vi "20_1.vi"() -> ()   [LabVIEW 2020]
uses:
  Tile/Tile.lvclass
  Tile/Set Tile ID.vi
  Tile/Set Tile.vi
  Tile/Get Matching Sides.vi
  <userlib>/_OpenG.lib/array/array.llb/Search 1D Array (U64)__ogtk.vi
  <userlib>/_OpenG.lib/array/array.llb/Index 1D Array Elements (U64)__ogtk.vi
panel:
  out "product":u64=8425574315321
  out "elements":u64[](array[numeric])=[1153, 1163, 1619, 3881]
  in  "Switch":bool
  in  "Input":string="Tile 3571:\n##..##....\n..##..#..#\n#...##....\n.....#...#\n..........\n...###....\n#......##.\n#...#...#.\n#...##...#\n#.####.##.\n\nTile 2687:\n#..##..###\n..........\n.....##..#\n.#.#..##.#\n#.#..#..##\n#.....#...\n#...#.....\n##....##..\n#...#...##\n..#.#.#.##\n\nTile 3049:\n##.#.#.###\n....##.###\n....##....\n#.........\n#.#...#..#\n#..##....#\n#.#......#\n#..#..##..\n#......###\n#.#..#...#\n\nTile 1597:\n###..##...\n##.....###\n.#..#..#.#\n#.......#.\n#.#.......\n.#..#.....\n#.....#...\n#........#\n##.#...##.\n.....#.###\n\nTile 1301:\n#.##.#.###\n#........#\n....#.....\n#.....####\n.#....#.##\n.....#....\n#..##..#.#\n.....#..##\n.#.##..#.#\n#...######\n\nTile 3259:\n..#####.#.\n.....#...#\n#...#.....\n...##...#.\n.#..#..##.\n.#.......#\n........##\n#.......#.\n.#.#...#..\n#...#.#..#\n\nTile 3989:\n#..#..####\n..........\n#........#\n.#....#...\n..........\n#.........\n.#........\n#........#\n...##.####\n.######.##\n\nTile 3803:\n#.####...#\n.###.#..#.\n....##..#.\n#........#\n..##..#...\n####.#....\n..#...#...\n#..#.....#\n..##....#.\n#....#...#\n\nTile 2897:\n.#..##.#.#\n..#.#...##\n#........#\n###.#..#.#\n...#..#.##\n...#....##\n....##...#\n.....##..#\n.#....#...\n..##....##\n\nTile 2843:\n##.###..##\n#.#.......\n#....#....\n#..##.##..\n.##..#.##.\n#....#....\n#.#...#.##\n..........\n.#...#...#\n###..#..##\n\nTile 3023:\n.#..###.#.\n.........#\n..........\n.#........\n#.#....#.#\n....#...#.\n#.......#.\n##.#.....#\n..#...#..#\n.....####.\n\nTile 2887:\n#....##...\n#...#.....\n##...##...\n#.....##.#\n.......#..\n#......#.#\n..##..#..#\n....#....#\n#.###.....\n#.####..#.\n\nTile 1013:\n#..####.#.\n#.##...#.#\n#..#..#...\n#..#..#..#\n...#......\n#.####...#\n.#..##..##\n...#.#..##\n....##..##\n#.##.#.#.#\n\nTile 3733:\n###.##.#.#\n..#....#..\n#...#.#..#\n....###..#\n.#........\n.....#....\n........##\n##........\n#........#\n#.#...#..#\n\nTile 3691:\n.##...####\n##..##....\n#.#.##..##\n#........#\n#.....##.#\n.....#....\n##.#.....#\n#..#.....#\n..#.......\n####....#.\n\nTile 3061:\n##.....#..\n.....#...#\n....##...#\n###.#.....\n#..#..###.\n#.#.###..#\n..#......#\n#..#.#...#\n..#.......\n..#.#..#..\n\nTile 1489:\n###.......\n.....##...\n..#...##..\n#.....#...\n#.#......#\n##.#..####\n...##.#...\n...#...#.#\n..........\n.##.##.#.#\n\nTile 1637:\n#########.\n.#.....#..\n#........#\n#........#\n.##.....##\n.........#\n#....#..##\n#.....####\n...###...#\n.#..##..##\n\nTile 1069:\n#.#...####\n##...#...#\n.....#...#\n.......##.\n......#..#\n#........#\n#...#.....\n......#...\n#.#..#....\n####.##.#.\n\nTile 1039:\n#..#######\n###.......\n.....#....\n#.........\n....#....#\n...####...\n.#...##...\n#.#....#.#\n........##\n#.#..#..#.\n\nTile 2767:\n.#.#..#.##\n.#..#....#\n#..#.#....\n#.#..##..#\n.####.#.##\n#....##...\n....##..##\n###.....#.\n..........\n....#.###.\n\nTile 2957:\n####.#####\n.......##.\n...#.....#\n...##..##.\n...##.##..\n#..#..#..#\n.....#....\n#..#....#.\n.##.......\n.##..#.##.\n\nTile 2789:\n.##..#.#.#\n#.#.....##\n#....#...#\n#....##...\n..#..#....\n#.........\n#.#..#..##\n#........#\n.#.......#\n#####...##\n\nTile 2837:\n.....#...#\n.....#.#.#\n#.......#.\n#...#...#.\n..#.....#.\n..#.#..#..\n##.......#\n....#....#\n#...#.....\n##.###....\n\nTile 3251:\n.######...\n...#......\n.#.#..###.\n#..#.##..#\n###.#....#\n#.#......#\n..#..###..\n##.#..#..#\n...#...###\n##.#..##..\n\nTile 3137:\n#####.#..#\n#.#..#.##.\n#.#..#....\n#.........\n.........#\n.........#\n...#......\n#...#...#.\n....#..#.#\n.#.###.#.#\n\nTile 3433:\n.##..####.\n...#......\n#..##....#\n....#....#\n#..###....\n..#......#\n.#..###...\n.##.#.....\n.........#\n.....#....\n\nTile 2551:\n#.########\n#.#.......\n##..#...##\n#.#..###.#\n#........#\n.#.#....#.\n#........#\n.##....#..\n#........#\n##..##.#..\n\nTile 2647:\n..####..##\n##....#..#\n#.........\n###.#.....\n#......#..\n....#...##\n.#..##.#.#\n.#.#..#...\n.....##.##\n.#.#...#..\n\nTile 1087:\n#..###..##\n#...#.#.#.\n.......#..\n..#.#.#..#\n#.......#.\n#....#....\n....#....#\n##...##..#\n#..#......\n.#..#.###.\n\nTile 1423:\n..#....#.#\n#........#\n.#.##.##..\n#.###.#.#.\n#.#......#\n...##...##\n#....#....\n....#....#\n.........#\n#####....#\n\nTile 1759:\n..#.#..#..\n##...#...#\n....#..#..\n#....#....\n.##..##..#\n...#.#...#\n#..#.....#\n##.......#\n......#..#\n#.##......\n\nTile 1583:\n.###.####.\n......###.\n......#..#\n.#...##...\n#...#....#\n..#.##....\n#...##..#.\n......#...\n#.....###.\n####.#....\n\nTile 1171:\n###......#\n#...##...#\n#####..##.\n#.......#.\n#.#...#..#\n#....#....\n....#....#\n##.....#.#\n#.#..#..##\n#.#.#..##.\n\nTile 2801:\n.###.####.\n......#...\n##..##.#.#\n.....#....\n#......#..\n###..##..#\n##.#..##.#\n#..#..#...\n#..#.#...#\n#..###.###\n\nTile 1559:\n.##..#...#\n#.##..#...\n...##..#..\n..#.#.....\n...#...#..\n.........#\n...#.....#\n#..##.#..#\n##..##....\n...###...#\n\nTile 2609:\n##.#..####\n..........\n#........#\n##.###...#\n#.#..#....\n..#..##..#\n#....#.#.#\n#.#.......\n#....#...#\n#.####.#.#\n\nTile 2287:\n#......#.#\n.....#.#.#\n..#..#...#\n##.#..#...\n..#..#.###\n.......###\n#......##.\n#.##.##...\n......#..#\n#####.##.#\n\nTile 3659:\n.###.#####\n#.#.......\n..........\n..#.....##\n#..#......\n#.#.#...##\n#.........\n.#...#....\n##.....#..\n#####.##.#\n\nTile 3539:\n.......#.#\n..##...#..\n.....#.#.#\n##.#......\n####......\n...#..#...\n#.......##\n#...#.....\n#..#.....#\n.##.#....#\n\nTile 3121:\n..##.#...#\n.###..#...\n##.#.#....\n#.....#..#\n#.#.......\n#.........\n....#...##\n......###.\n#........#\n#..###..##\n\nTile 2237:\n...##.....\n..........\n...#......\n#....#...#\n#.........\n.......#..\n#...###..#\n.....#...#\n.........#\n#.####.##.\n\nTile 1277:\n.###...##.\n.......###\n#.....##..\n#.##..###.\n#.#..#....\n.....#....\n#...#....#\n#.#......#\n#...###..#\n...##...##\n\nTile 2161:\n..#####..#\n#....##..#\n#.....#..#\n....#....#\n.....#.##.\n..........\n#......#.#\n#..#......\n#....#..##\n.##.....#.\n\nTile 3709:\n.#..#...##\n#..#.....#\n...#....#.\n..........\n.#...#....\n..........\n....##....\n#.........\n.........#\n..####....\n\nTile 1117:\n##.##.#..#\n.....##...\n.#.#..#.##\n.#...#..#.\n#.##.#....\n####.....#\n##..#.....\n#.........\n#...##...#\n####..#.#.\n\nTile 2081:\n##.##.###.\n#...#.....\n#.....#...\n#.#..#.#..\n#.....#..#\n...#.....#\n#....#....\n......#..#\n.#.##..#..\n###..#.#.#\n\nTile 1709:\n##...#.##.\n###..#....\n#.......#.\n#.....##..\n.........#\n#....#..##\n..#...##..\n#...#.....\n#...#.#..#\n.###.#....\n\nTile 2927:\n...###..##\n##.#......\n..........\n##........\n#....#...#\n.......##.\n#.....#..#\n##.#.#....\n#......#..\n...#.####.\n\nTile 1499:\n#....##.#.\n......#...\n#........#\n......#...\n.#.......#\n#.#...#.##\n..#....#.#\n#...#.....\n.........#\n#.....##.#\n\nTile 1453:\n#.##.####.\n..#...##..\n.........#\n.........#\n#..#..#...\n.........#\n#....#.#..\n#.....#..#\n.#........\n#....#....\n\nTile 1283:\n.#.##..###\n..#...#.#.\n...##..#..\n#.......#.\n#......#..\n#..##.....\n#.......##\n....##...#\n..#.....##\n##.#.#...#\n\nTile 2063:\n......#.##\n.........#\n....##..#.\n.#....##..\n##........\n.###.###.#\n#.#....#..\n....#...#.\n#......###\n#....####.\n\nTile 3529:\n...###.##.\n#....#...#\n...#.....#\n...#.#..#.\n.#.#.....#\n#...#.....\n##..#..#..\n#.....#..#\n.#........\n.#..#####.\n\nTile 2657:\n..#.##..#.\n##..#...##\n#.....#...\n#....##...\n.....#..##\n#.#..##.##\n#.........\n#.#...##.#\n##....#...\n##..####.#\n\nTile 2089:\n.#########\n##.#.##..#\n#........#\n#..###..##\n...#......\n##..#....#\n#...#..#..\n#..#....#.\n..#.#....#\n...###...#\n\nTile 3779:\n#.#...##.#\n.##...##..\n.....##...\n.#....##.#\n###..##..#\n#.#..#.#..\n....##...#\n##...#....\n.#...#....\n#######...\n\nTile 3217:\n...##.....\n....##....\n.....##..#\n##...#.#.#\n###.......\n...#...#..\n...#.....#\n#..#.#.###\n##.#...#.#\n.#.#..##..\n\nTile 3907:\n..#..##.##\n#.#.....##\n#.......#.\n.#...###..\n..###.####\n##.#..##..\n#.........\n##...#..#.\n#....#....\n.#.....#.#\n\nTile 3547:\n#..#.##...\n#..###...#\n##.......#\n.....#....\n#...#...#.\n#..#..#...\n........#.\n......##.#\n.......#..\n.##.#..##.\n\nTile 3187:\n##.#.##...\n#...#.##.#\n#...#.....\n#....#..##\n....#.#..#\n.....#....\n.....#..##\n....##...#\n..........\n#######.##\n\nTile 1217:\n##.#####..\n#.......#.\n...#....##\n#........#\n#.#......#\n.....#...#\n#.........\n....#...##\n#...#.....\n.#...###.#\n\nTile 3821:\n#.###.###.\n#.#......#\n#..#.#...#\n.##...#.##\n...#....##\n#...#..##.\n#......#.#\n###..#...#\n.........#\n#....##.##\n\nTile 1607:\n##..#..##.\n#.##....##\n###.##.##.\n.#....##.#\n#.#..#...#\n.....#.#..\n#.#..#..#.\n#.#..#....\n..........\n......##.#\n\nTile 1459:\n.###.##..#\n#.......#.\n##........\n..#...####\n###.......\n#....#....\n.#.....#.#\n###..#..##\n.....#....\n..#..#..##\n\nTile 2129:\n....#.#..#\n#.....##.#\n#........#\n..........\n..#......#\n#.....#..#\n.#..##...#\n#.#.#..#.#\n#.........\n#.##....##\n\nTile 1601:\n.#.#.#.#.#\n..#..##...\n#.#.#...#.\n....##....\n....##.#..\n..#.......\n#.....#..#\n#..##.#...\n.........#\n...####.#.\n\nTile 1801:\n#.#...#.#.\n..#....#..\n#..#...#..\n......#...\n.....#....\n#.#..##.##\n#.........\n...#.#...#\n.#....#..#\n#.....##..\n\nTile 2447:\n..#.....##\n.#..#...##\n.....#.#..\n.#....#..#\n#...####.#\n##.##..###\n.#.......#\n#.##.....#\n#.......##\n.###.#...#\n\nTile 2203:\n#.....##..\n#.#.......\n........##\n###...#...\n..........\n#..#.....#\n....#.##.#\n..##.....#\n.#...#...#\n#.###..#..\n\nTile 1381:\n.#...#...#\n....#.....\n##.......#\n#.....#...\n.........#\n.#.......#\n.......##.\n#.#.....##\n.#..#.##..\n##.#.##.#.\n\nTile 3163:\n#...####.#\n#......##.\n...###.#.#\n#....##...\n#......###\n.....#..##\n.#..###...\n#..##..#..\n#.....#...\n#.#####.##\n\nTile 3673:\n.#....##.#\n..#..####.\n#.....#...\n...#....#.\n#....#...#\n#....##.#.\n##...#.#..\n.#..#.#...\n#..#.....#\n####.##...\n\nTile 3919:\n....##.##.\n##..##....\n...##...##\n#...#.....\n..........\n....#..###\n.#.....#..\n....#..#.#\n.##..#....\n.#...###.#\n\nTile 2437:\n..##...#.#\n#....#...#\n#..#.....#\n..#.#...##\n.......#..\n........##\n........##\n.......#.#\n#....#.#.#\n##..#.###.\n\nTile 2969:\n##.#.##.#.\n#.##....#.\n.##......#\n#.#.#....#\n#.#.......\n.........#\n....#.#.##\n.#.......#\n...#..#.##\n##.#.##..#\n\nTile 2621:\n.##.##.#..\n.##...#...\n..........\n#.........\n#.#.#.#..#\n..#..#...#\n.......#.#\n#.#.....##\n...#..#...\n#.......##\n\nTile 3613:\n##..#....#\n#..##.....\n..#.......\n..#...#...\n...#...#..\n...#.....#\n..#.....#.\n..#.###..#\n..........\n..#.####..\n\nTile 2777:\n##.#####.#\n#.##.#...#\n..#.......\n.##...##.#\n.........#\n.#.###.##.\n#......##.\n#......##.\n#...##..##\n#..#....##\n\nTile 2711:\n#..#..##..\n..........\n#.#......#\n#.....####\n..........\n##.......#\n........#.\n#.......#.\n#.#..#...#\n#.#.####.#\n\nTile 2281:\n.#.###...#\n###....#..\n..........\n#.#..#..##\n.........#\n###..#.##.\n####..#..#\n##..#.....\n##..#..#..\n#.....#..#\n\nTile 1579:\n....#..#..\n#........#\n#...#..#..\n..##.#.#..\n.###.#...#\n....##..#.\n...##.#...\n.#.##....#\n.#.......#\n##...#...#\n\nTile 2411:\n#.#....##.\n..#...#..#\n.#..##....\n.#..##...#\n.....#.#.#\n......##..\n#.#....###\n.#.##....#\n..#..#....\n..#.###..#\n\nTile 2963:\n.......##.\n.....#....\n.........#\n#.....#..#\n.....#.#..\n.....#.##.\n.#.#...###\n#.#.......\n.#.......#\n###..#..#.\n\nTile 1693:\n#.##..##..\n..........\n.........#\n.##..#...#\n.........#\n#........#\n###......#\n..#...#...\n.#.##....#\n...#.#...#\n\nTile 2399:\n###.#.##..\n#...#.....\n...#...#.#\n###.......\n.##.##....\n##.....#.#\n####......\n##.......#\n#..#...#.#\n#...#.....\n\nTile 1913:\n##.....###\n........##\n#.....###.\n..........\n....#...#.\n#.#.....#.\n#....#...#\n..#...#...\n....#..#..\n#..####...\n\nTile 3343:\n.....#.##.\n..#...#...\n####.....#\n....#.....\n......#..#\n......#...\n#........#\n#.......#.\n..#...#.#.\n.....###.#\n\nTile 2557:\n#.......##\n....#...##\n#......#.#\n#.#.#.#.##\n#..##.....\n..###.#.#.\n#..#......\n#...#.....\n....#....#\n#.##...#.#\n\nTile 1097:\n.#.#.#..##\n..#.#.....\n##........\n.##...##..\n..#..#...#\n#........#\n........##\n#.#.#.....\n.#.#.....#\n#.##..#...\n\nTile 2591:\n##..#..###\n......#...\n...###.#..\n#.......#.\n#.#.....#.\n#.##..#...\n....##.#..\n#.#..#...#\n#.###..#.#\n##........\n\nTile 3413:\n...##...##\n..#....#..\n##.#....#.\n#..#....#.\n#........#\n#..#......\n#.....#.##\n##.....#.#\n#....#....\n####.#...#\n\nTile 2087:\n###..###.#\n##......#.\n#..#...#.#\n#.#.......\n##.#.....#\n#.#.#.....\n...#.....#\n..........\n#.........\n#.##..###.\n\nTile 3037:\n......##..\n..#..#....\n#.#.......\n#.#....#..\n.#.#.##..#\n#.....#.##\n#.....#.#.\n.#..##...#\n#....##...\n...#..###.\n\nTile 2239:\n.####..#..\n#.........\n.#.......#\n#..##.....\n##..##..##\n#.#....#..\n.........#\n#.......#.\n....#.....\n#.###..#.#\n\nTile 3313:\n##.##.#..#\n.#.#..#...\n.##...##.#\n.#.##..#..\n##........\n..........\n#..#.#....\n#.........\n..........\n.##..#..#.\n\nTile 3361:\n.###.#...#\n##..#.#..#\n...##....#\n#..##.....\n..........\n#......#.#\n.........#\n..#..##.#.\n#..#...###\n#...#.#.#.\n\nTile 3167:\n..##..####\n#.....#.#.\n.....#.#..\n...#......\n....#.#.##\n...#.#.#..\n.......#..\n##........\n#..#...#.#\n####.##..#\n\nTile 1979:\n#.#.###...\n..#.....##\n...#...##.\n#.......##\n........##\n..##..#...\n..#......#\n#.#....#.#\n#..#.....#\n.##.......\n\nTile 1831:\n##.##.##.#\n#.........\n.........#\n##.......#\n###.....##\n..##..##..\n##.....#.#\n#....#...#\n###.##..#.\n#..#####..\n\nTile 1487:\n#..#....##\n.#..#....#\n#....#....\n#.........\n#.#...#.##\n#..##...##\n...##..#..\n.#...##...\n.#........\n.#...#..#.\n\nTile 1987:\n###..#....\n##..##...#\n......#..#\n.#.#...#.#\n.....#.#..\n....#..#..\n....###..#\n#...##....\n###.....#.\n...##.####\n\nTile 3083:\n....##..#.\n##..#.###.\n#..#...##.\n#.###.....\n.........#\n....#.....\n.#........\n.#........\n#.........\n#.#.#.##.#\n\nTile 1543:\n...##..###\n.........#\n.......#.#\n#..#..#.##\n##....#.#.\n....#..#..\n#..#......\n...#...#.#\n##.##..#..\n#.###..#..\n\nTile 1151:\n#.#..#####\n#.#..#...#\n#..#......\n....#...#.\n..........\n#...#.#..#\n#..#.#...#\n##....#..#\n#.........\n##.....###\n\nTile 1009:\n##..#...##\n#....#...#\n.#...#....\n#........#\n.#..#..#..\n.###.##.#.\n#......#.#\n##.#..##..\n#....#.###\n####...##.\n\nTile 3929:\n......#.#.\n#..#.##.##\n....#.#.##\n#.##..#...\n###..#..#.\n.##..###.#\n.##......#\n....#....#\n........#.\n.#...###..\n\nTile 1321:\n#.##..#...\n.##.....##\n#.#..#....\n...#.....#\n###......#\n#.#.#.##.#\n##.......#\n##......#.\n.#...#....\n.#..##..##\n\nTile 2017:\n###.#..###\n.#..###..#\n#..#......\n.........#\n..#...##..\n....#.##.#\n...##.#..#\n....#...##\n#..#..##..\n##.#.#.#..\n\nTile 1747:\n....##.#..\n#........#\n.....#..#.\n..#####...\n######..#.\n##..#.#...\n.###..#..#\n#.....#...\n.##..#..##\n..#####...\n\nTile 3089:\n#....#.##.\n#.....#..#\n..........\n#..#.#....\n.......#..\n#.....#...\n........#.\n##..#..##.\n#.....#..#\n#.#.#....#\n\nTile 3019:\n.#..###.##\n.#...#...#\n#.#.......\n###.......\n#....#...#\n#.##...#..\n##........\n.#.......#\n.#.#......\n.#..#...#.\n\nTile 3079:\n...#.###..\n#......#..\n#.......##\n#...#..###\n#.......#.\n......#.#.\n#........#\n.#.#...###\n..#.#....#\n...#...#.#\n\nTile 1663:\n##.##..###\n#.....##.#\n......#.##\n#........#\n..#.#.....\n....#..#.#\n#.#.#..#.#\n#.......#.\n..#......#\n#.#..#....\n\nTile 1823:\n.###...###\n#.#.#..##.\n..........\n.........#\n###....#..\n..........\n##....#.##\n#.......##\n..#..#...#\n......####\n\nTile 3823:\n....#..#..\n..#.#..#.#\n###.#.##.#\n..##....#.\n#.........\n#....#...#\n#.......##\n#.#...##..\n..#....#..\n..#....##.\n\nTile 1901:\n#.#.#....#\n..#....#.#\n...#..#.#.\n.#..#..###\n....####..\n......#...\n#....#....\n..#....#..\n#......#..\n######.#..\n\nTile 3347:\n#.#.....#.\n#..#..#...\n#.#.......\n#..#.#....\n...#......\n#.........\n##.#.....#\n#........#\n#....#...#\n#.#.##.###\n\nTile 1873:\n..###.#.##\n.#.#....#.\n#........#\n..#..#...#\n##.....#..\n#........#\n#.........\n.#........\n#.#..#.#.#\n.##.#...##\n\nTile 2053:\n#.#.#.#..#\n#...###..#\n##.##.##.#\n....##.#.#\n#.###....#\n#.....#..#\n#..##.####\n....#..#..\n#.........\n#..#.#..#.\n\nTile 2659:\n.#....##.#\n#.#......#\n#..#......\n.#.###.#.#\n..........\n#........#\n.......#.#\n....#....#\n#........#\n##..##.#..\n\nTile 2503:\n.#..####.#\n#.##......\n..#....###\n..#..#.###\n...##...##\n..#.....#.\n..........\n##.#......\n#.#.......\n#...#..#.#\n\nTile 3881:\n##.###.###\n#......#..\n#...#....#\n..#.#....#\n#..#..#..#\n#..#.....#\n...#..##.#\n#.#.......\n#..##....#\n...#.##...\n\nTile 1973:\n..#.###.#.\n#.##....##\n#.......##\n##......##\n#.........\n#.#..#....\n.#....###.\n..#.#..#..\n......#..#\n#..#.....#\n\nTile 3329:\n.#.#.###.#\n..#.#.....\n.#.......#\n#..#.##.##\n#.##..####\n..#.##..##\n....#.....\n#...#.#.#.\n...#.#...#\n.#...##..#\n\nTile 3331:\n#......###\n#......#.#\n#.#.#.#..#\n........#.\n.##.####..\n#..#..#..#\n.#.......#\n......#.##\n......#.#.\n.##...#.#.\n\nTile 1307:\n##.#.#..#.\n.........#\n.#....##.#\n#.........\n#.........\n#....#.#..\n........##\n......##..\n..#.##...#\n..##...##.\n\nTile 2543:\n.#.#.##.##\n#........#\n..##......\n#.........\n##...#...#\n.###..##.#\n.##......#\n.#........\n.....#.#..\n...######.\n\nTile 2003:\n#.#..#.#.#\n.....#....\n#.#.#.....\n####.#..##\n..###....#\n....#.#...\n#.####...#\n.##...#.##\n#.#.#..#..\n...#.....#\n\nTile 3301:\n##....##.#\n.....#...#\n#........#\n..........\n###.##.#..\n.....#...#\n#.#......#\n....##...#\n#........#\n.#.#...#.#\n\nTile 2297:\n#..#.##..#\n...#.#.##.\n..###..#..\n##..#.....\n####..#..#\n..#.#..#..\n.....#...#\n#...#.....\n#.....#..#\n##....#...\n\nTile 2311:\n##.....#.#\n##........\n#........#\n#...##....\n#......#..\n.........#\n.........#\n#..#.#....\n.....#...#\n###.#..##.\n\nTile 1361:\n.#.##.#..#\n#.#..#...#\n#....###..\n..###.#...\n#..#.....#\n#..#...##.\n#.#.....#.\n.......#.#\n##.##.....\n#.###.#..#\n\nTile 1481:\n.####.#.##\n..........\n.........#\n###.#.#...\n##....##.#\n..#...#.##\n..##.#.#..\n#.#.....##\n.......#..\n....###...\n\nTile 1153:\n.##.##..##\n###......#\n#....##...\n......#.#.\n#....#....\n.....##..#\n.....#...#\n#.........\n#...#....#\n##..#.#...\n\nTile 2153:\n#.###.#..#\n..#.##....\n..##....#.\n##...#...#\n#...#.....\n........#.\n#..##...#.\n..#.......\n#...##.#..\n#.#.#.#...\n\nTile 2377:\n.##..##.#.\n...##..#.#\n#.#.#.....\n#.##......\n#.....#..#\n#...#....#\n...##....#\n...###....\n.#.##...##\n.###.##...\n\nTile 3863:\n.##.###.##\n.......#.#\n#........#\n##.#.#...#\n##...#...#\n#...##....\n#..#..#.##\n.....#####\n##.#..###.\n....###...\n\nTile 1163:\n##..######\n#........#\n.#.#...###\n..#..#...#\n##..#...##\n#.#.......\n#.#..#....\n#..#.#....\n###..#...#\n.#####.###\n\nTile 2207:\n.#..#.#.##\n##.....#.#\n#..#.....#\n#..#....##\n.........#\n...#.....#\n#...#..#..\n..#.....##\n.....#....\n#.##.....#\n\nTile 1201:\n#.##.##..#\n#.#.......\n#..#.....#\n.###...#..\n#.#......#\n........##\n.........#\n.##....#.#\n..##.#...#\n.......###\n\nTile 1619:\n#.....#.#.\n...#.##..#\n#.....#...\n#...#.....\n#..#...#.#\n#..##.#...\n.#...#.#..\n#......##.\n#.........\n#.##...###\n\nTile 3389:\n...#..##..\n#........#\n#...#.....\n#.#....#.#\n###....#.#\n#.#....###\n#..##..#.#\n.##.#.#..#\n#...###...\n#...#....#\n\nTile 3359:\n.###..##..\n#........#\n###...#.#.\n........##\n....#..#.#\n.#.#......\n#........#\n.......#.#\n.#.....#..\n##.###....\n"
  in  "Input Test":string="Tile 2311:\n..##.#..#.\n##..#.....\n#...##..#.\n####.#...#\n##.##.###.\n##...#.###\n.#.#.#..##\n..#....#..\n###...#.#.\n..###..###\n\nTile 1951:\n#.##...##.\n#.####...#\n.....#..##\n#...######\n.##.#....#\n.###.#####\n###.##.##.\n.###....#.\n..#.#..#.#\n#...##.#..\n\nTile 1171:\n####...##.\n#..##.#..#\n##.#..#.#.\n.###.####.\n..###.####\n.##....##.\n.#...####.\n#.##.####.\n####..#...\n.....##...\n\nTile 1427:\n###.##.#..\n.#..#.##..\n.#.##.#..#\n#.#.#.##.#\n....#...##\n...##..##.\n...#.#####\n.#.####.#.\n..#..###.#\n..##.#..#.\n\nTile 1489:\n##.#.#....\n..##...#..\n.##..##...\n..#...#...\n#####...#.\n#..#.#.#.#\n...#.#.#..\n##.#...##.\n..##.##.##\n###.##.#..\n\nTile 2473:\n#....####.\n#..#.##...\n#.##..#...\n######.#.#\n.#...#.#.#\n.#########\n.###.#..#.\n########.#\n##...##.#.\n..###.#.#.\n\nTile 2971:\n..#.#....#\n#...###...\n#.#.###...\n##.##..#..\n.#####..##\n.#..####.#\n#..#.#..#.\n..####.###\n..#.#.###.\n...#.#.#.#\n\nTile 2729:\n...#.#.#.#\n####.#....\n..#.#.....\n....#..#.#\n.##..##.#.\n.#.####...\n####.#.#..\n##.####...\n##..#.##..\n#.##...##.\n\nTile 3079:\n#.#.#####.\n.#..######\n..#.......\n######....\n####.#..#.\n.#...#.##.\n#.#####.##\n..#.###...\n..#.......\n..#.###..."
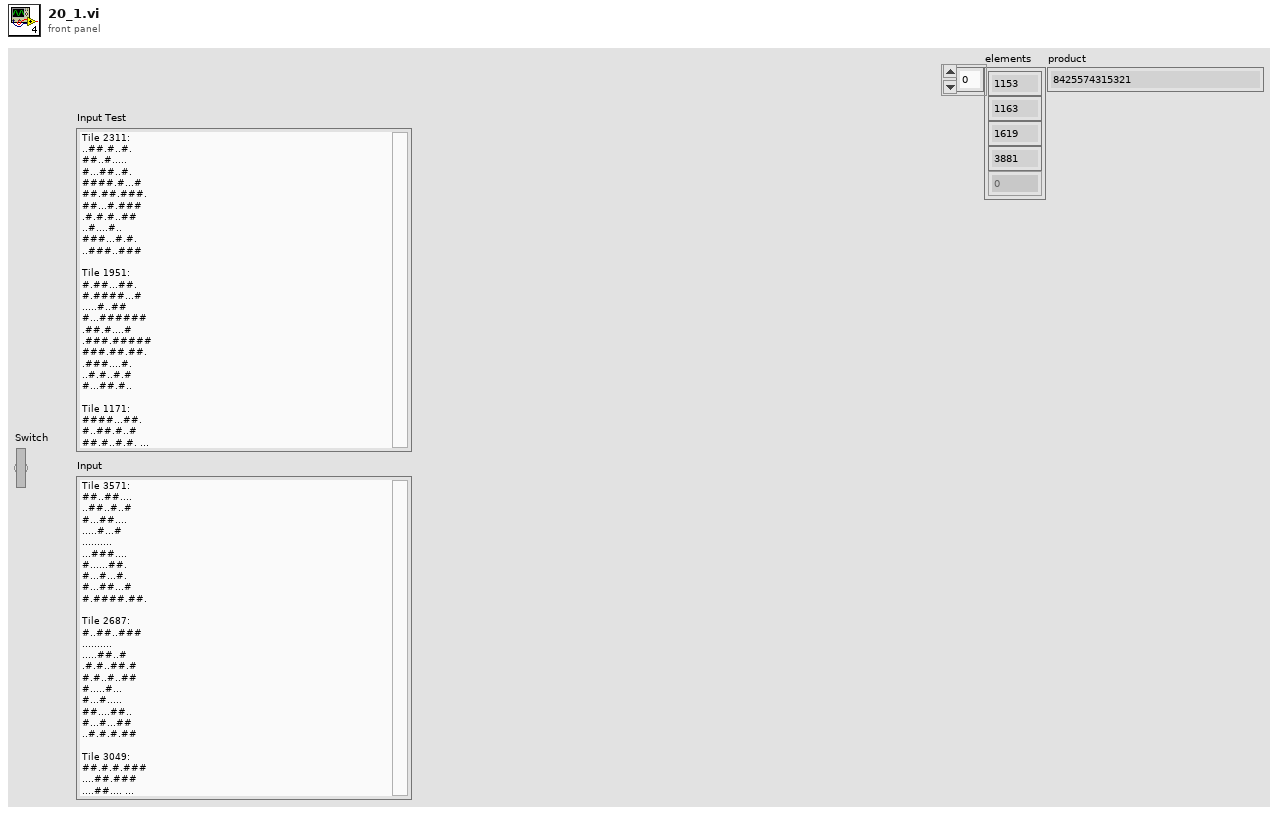
[diagram p1: front panel]
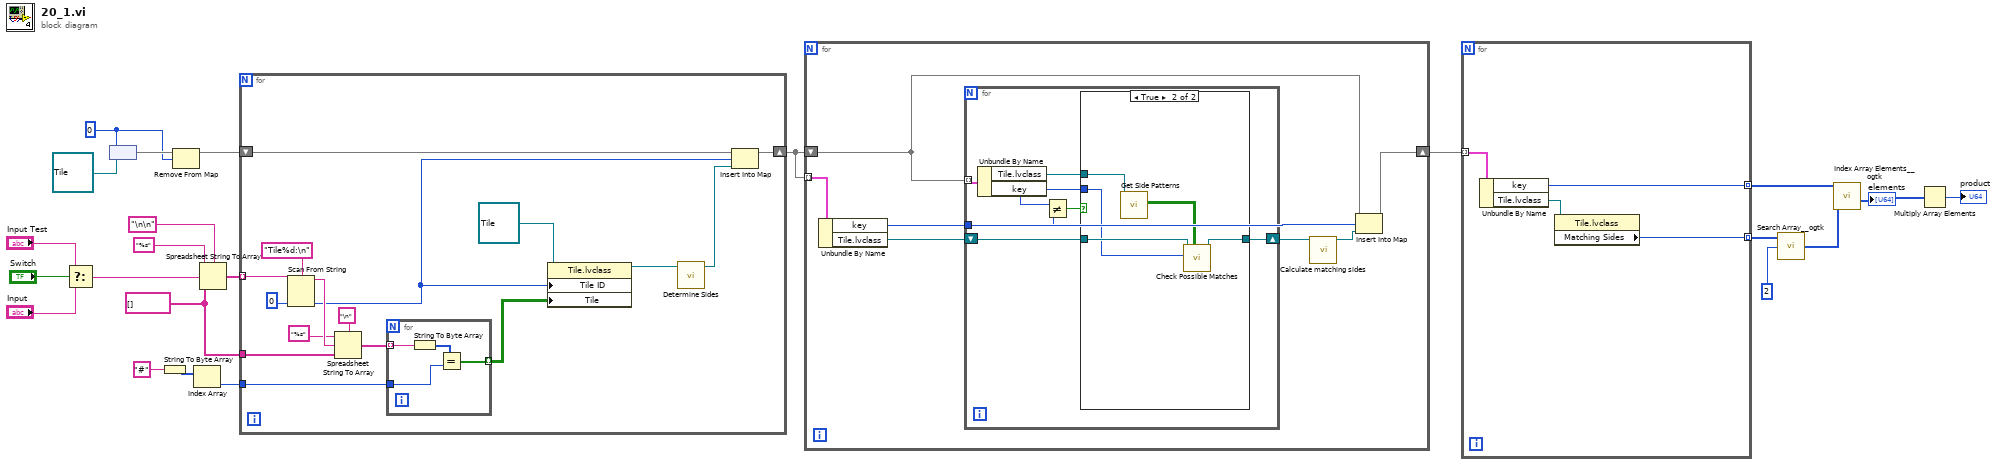
[diagram p0: block diagram]
diagram:
  w18 = u64 0
  w13 = string[] []
  n1 = Select(t="Input Test", s="Switch", f="Input") -> (s? t:f=w9:string)
  n2 = node(w18, refnum<class "Tile.lvclass"> refnum ("Tile.lvclass")) -> (w20:map{u64, refnum<class "Tile.lvclass">})
  n3 = String To Byte Array(string="#") -> (unsigned byte array=w16:u8[])
  n4 = Remove From Map(10:w18, 11:w20) -> (3:w19:map{u64, refnum<class "Tile.lvclass">})  [unwired: 2 out]
  n5 = Index Array(array=w16) -> (element=w14:u8)  [unwired: 1 in]
  n6 = Spreadsheet String To Array(delimiter (Tab)="\n\n", format string="%s", spreadsheet string=w9, array type (2D Dbl)=w13) -> (array=w21:string[])
  n7 = for {
    tunnel: w21 -> [w37] mode=indexing
    shift-right: [w34] -> w8
    shift-left: w19 -> [w38]
    tunnel: w14 -> [w33]
    tunnel: w13 -> [w29]
    n8 = Scan From String(format string="Tile%d:\n", input string=w37, default 1=u64 0) -> (remaining string=w31:string, output 1=w24:u64)  [unwired: 2 in, 2 out]
    n9 = Spreadsheet String To Array(delimiter (Tab)="\n" ("format string"), format string="%s", spreadsheet string=w31, array type (2D Dbl)=w29) -> (array=w28:string[])
    n10 = for {
      tunnel: w33 -> [w43]
      tunnel: w28 -> [w42] mode=indexing
      tunnel: [w40] -> w27 mode=indexing
      n11 = String To Byte Array(string=w42) -> (unsigned byte array=w41:u8[])
      n12 = Equal?(x=w41, y=w43) -> (x = y?=w40:bool[])
    }
    n13 = property class="Tile.lvclass"(reference=refnum<class "Tile.lvclass"> refnum ("Tile.lvclass"), "Tile ID"=w24, "Tile"=w27) -> (reference out=w26:refnum<class "Tile.lvclass">)  [unwired: 1 in, 1 out]
    n14 = call "Determine Sides.vi"("Tile in"=w26) -> ("Tile out"=w25:refnum<class "Tile.lvclass">)  [unwired: 9 in, 1 out]
    n15 = Insert Into Map(map in=w38, key=w24, value=w25) -> (map out=w34:map{u64, refnum<class "Tile.lvclass">})  [unwired: 2 out]
  }
  n16 = for {
    shift-right: [w49] -> w7
    shift-left: w8 -> [w47]
    tunnel: w8 -> [w50] mode=indexing
    n17 = Unbundle By Name(w50) -> ("key"=w48:u64, "Tile.lvclass"=w46:refnum<class "Tile.lvclass">)
    n18 = for {
      tunnel: w47 -> [w57] mode=indexing
      tunnel: w48 -> [w53]
      shift-right: [w51] -> w45
      shift-left: w46 -> [w52]
      n19 = Unbundle By Name(w57) -> ("Tile.lvclass"=w56:refnum<class "Tile.lvclass">, "key"=w54:u64)
      n20 = Not Equal?(x=w54, y=w53) -> (x != y?=w55:bool)
      n21 = case shown="True" w55 {
        tunnel: w56 -> [_ w63]
        tunnel: w54 -> [_ w60]
        tunnel: w52 -> [w58 w62]
        tunnel: [w58 w59] -> w51
        frame False {
        }
        frame True {
          n22 = call "Get Side Patterns.vi"("Tile in"=w63) -> ("Sides"=w61:bool[][])  [unwired: 8 in, 2 out]
          n23 = call "Check Possible Matches.vi"("Patterns In"=w61, "ID In"=w60, "Tile in"=w62) -> ("Tile out"=w59:refnum<class "Tile.lvclass">)  [unwired: 7 in, 1 out]
        }
      }
    }
    n24 = call "Calculate matching sides.vi"("Tile in"=w45) -> ("Tile out"=w44:refnum<class "Tile.lvclass">)  [unwired: 9 in, 1 out]
    n25 = Insert Into Map(map in=w47, key=w48, value=w44) -> (map out=w49:map{u64, refnum<class "Tile.lvclass">})  [unwired: 2 out]
  }
  n26 = for {
    tunnel: w7 -> [w67] mode=indexing
    tunnel: [w65] -> w4 mode=indexing
    tunnel: [w64] -> w6 mode=indexing
    n27 = Unbundle By Name(w67) -> ("key"=w65:u64, "Tile.lvclass"=w66:refnum<class "Tile.lvclass">)
    n28 = property class="Tile.lvclass"(reference=w66) -> ("Matching Sides"=w64:u64)  [unwired: 1 in, 2 out]
  }
  n29 = call-poly <userlib>:"Search Array__ogtk.vi"("Array"=w6, "Element Data"=u64 2 ("Matching Sides")) -> ("Indices of Elements"=w3:i32[])  [unwired: 7 in]
  n30 = call-poly <userlib>:"Index Array Elements__ogtk.vi"("indices"=w3, "array"=w4) -> ("elements"=w2:u64[])  [unwired: 9 in]
  "elements" <- w2
  n31 = Multiply Array Elements(1:w2) -> (0:→"product":u64)
